vi "table test test.vi"() -> ()   [LabVIEW 2019]
uses:
  Ctrl/Table Save.ctl
  Ctrl/MeasureDisplayTab.ctl
  Ctrl/PD Table Save Low Index.ctl
  Ctrl/PD Table Save Col Index.ctl
  <vilib>/Utility/sysdir.llb/System Directory Type.ctl
  <vilib>/Utility/file.llb/Read Delimited Spreadsheet (string).vi
  <vilib>/Utility/file.llb/Write Delimited Spreadsheet (string).vi
panel:
  in  "SN":string="012345678911111111112"
  out "硬體":string
  out "Read SN Table":string[][](array[string])
  out "first row":string[](array[string])
  out "all rows":string[][](array[string])
  out "error out":errorcluster
  in  "Read SN Table 2":string[][](array[string])
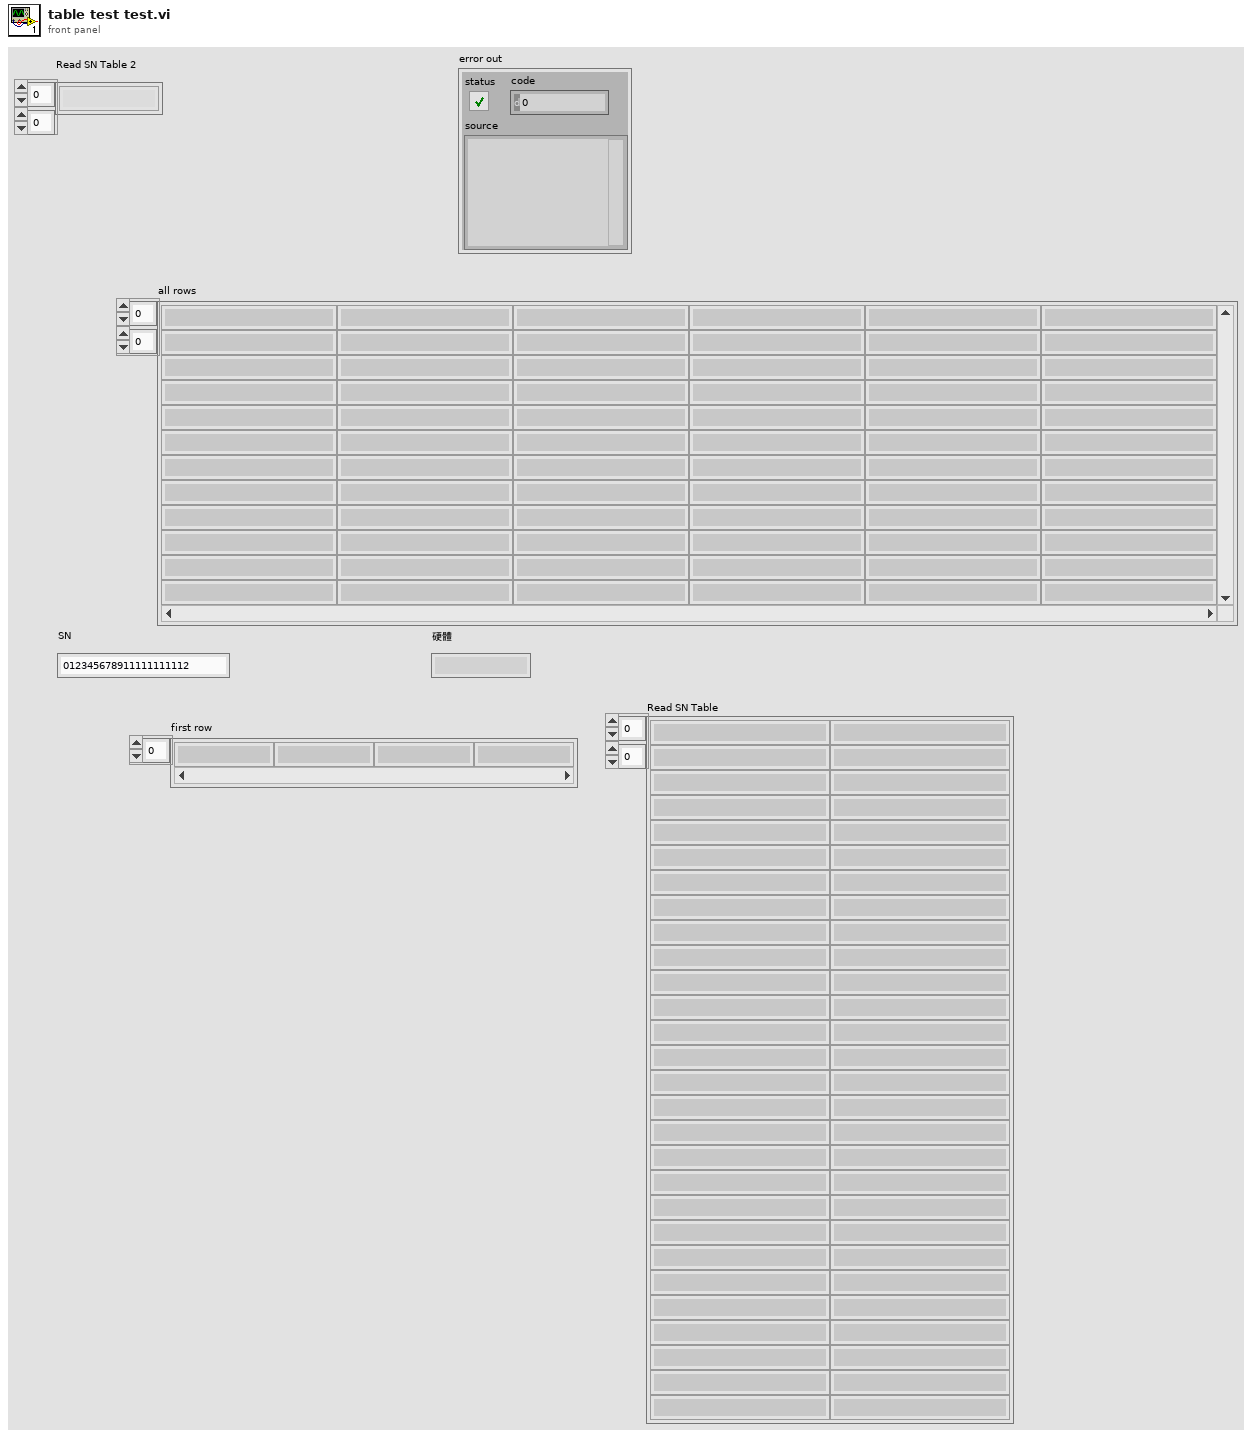
[diagram p1: front panel]
types:
  T1 = typedef "Table Save.ctl" = enum16{"initial", "Add", "Write", "Replace", "Delete", "REad", "RedTable", "Load"}
  T2 = typedef "MeasureDisplayTab.ctl" = enum16{"Tray Barcode", "PCBA BARCODE", "硬體(Tool初始化)", "company(Tool初始化)", "耗電流 uA(電流表)", "電池負載電壓", "晶片ID(Tool FORMAT)", "雷雕ID(TOOl scan、藍芽接收器)", "Format(Tool FORMAT)", "Programe(Tool Programe)", "MAC(藍芽接收器)", "ID(藍芽接收器)", "KPA(藍芽接收器)", "溫度(藍芽接收器)", "SENSOR電池電壓(藍芽接收器)", "RSSI(藍芽接收器)", "SensorType_315(FSK scan)", "FSKsnVol_315(FSK scan)", "FSKscanl_315(FSK scan)", "P_315(FSK scan)", "T_315(FSK scan)", "SensorType_433(ASK scan)", "ASKsnVol_433(ASK scan)", "ASKscan_433(ASK scan)", "P_433(ASK scan)", "T_433(ASK scan)", "測高Data"}
  T3 = typedef "PD Table Save Col Index.ctl" = enum16{"Col A", "Col B", "PCBA SN_C", "scan 半成品 ID_1_D", "半成品 Waste_Time_E", "半成品 Result_F", "半成品 DateTime_G", "433半成品 版本_H", "433半成品 company_I", "433半成品 FF_J", "433半成品 SensorType_K", "433半成品 BattVol_L", "433半成品 ASKsnVOL_M", "433半成品 ID_2_N", "433半成品 Format_O", "433半成品 Programe_P", "433半成品 ASKscan_Q", "433半成品 FSKscan_R", "433半成品 Batt_S", "433半成品 SN_T", "433半成品 Ptest_U", "433半成品 Ttest_V", "433半成品 P_W", "433半成品 T_X", "433半成品 結果_Y", "433半成品 箱號_Z", "不良代碼_AA", "電流_AB", "電池電壓_AC", "315半成品 版本_AD", "315半成品 company_AE", "315半成品 FF_AF", "315半成品 SensorType_AG", "315半成品 BattVol_AH", "315半成品 ASKsnVOL_AI", "315半成品 ID_2_AJ", "315半成品 Format_AK", "315半成品 Programe_AL", "315半成品 ASKscan_AM", "315半成品 FSKscan_AN", "315半成品 Batt_AO", "315半成品 SN_AP", "315半成品 Ptest_AQ", "315半成品 Ttest_AR", "315半成品 P_AS", "315半成品 T_AT"}
  T4 = typedef "PD Table Save Low Index.ctl" = enum16{"low 1", "low 2", "low 3", "low 4", "一般模式F", "一般模式P", "一般模式S", "low 8", "藍芽模式F", "藍芽模式P", "藍芽模式S"}
  T5 = typedef "System Directory Type.ctl" = i32
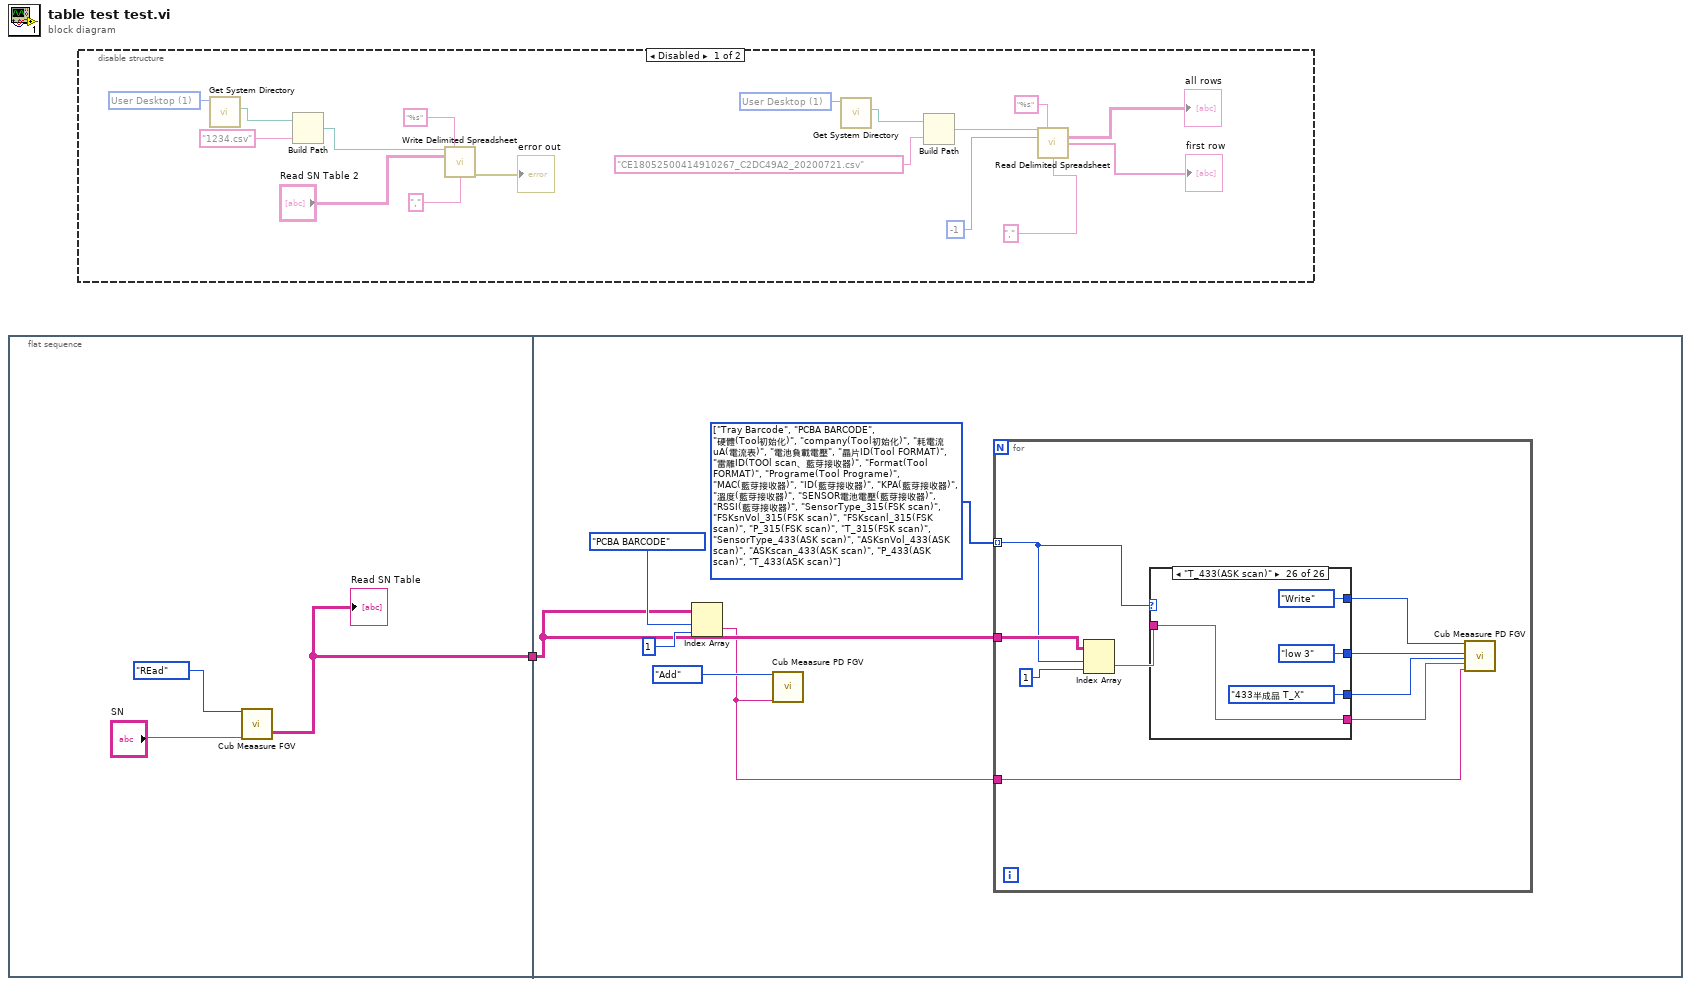
[diagram p0: block diagram]
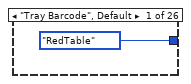
[diagram p3: hidden frame]
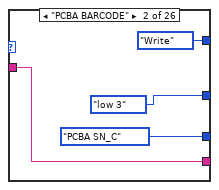
[diagram p4: hidden frame]
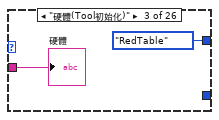
[diagram p5: hidden frame]
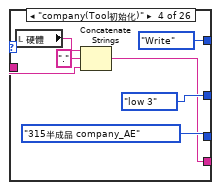
[diagram p6: hidden frame]
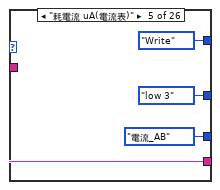
[diagram p7: hidden frame]
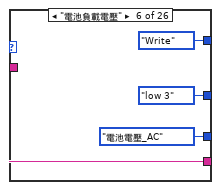
[diagram p8: hidden frame]
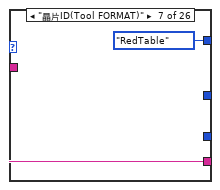
[diagram p9: hidden frame]
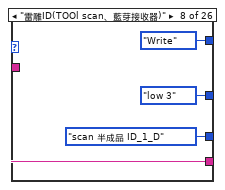
[diagram p10: hidden frame]
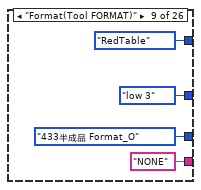
[diagram p11: hidden frame]
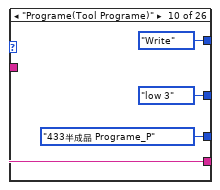
[diagram p12: hidden frame]
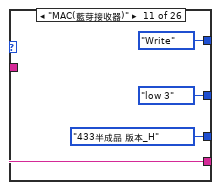
[diagram p13: hidden frame]
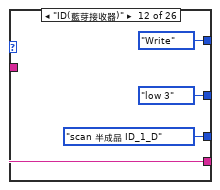
[diagram p14: hidden frame]
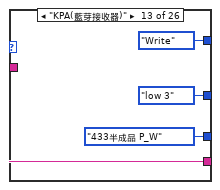
[diagram p15: hidden frame]
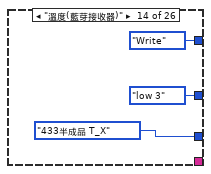
[diagram p16: hidden frame]
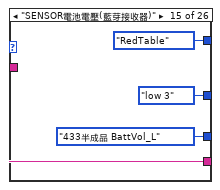
[diagram p17: hidden frame]
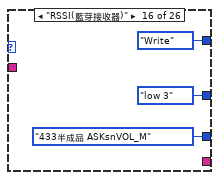
[diagram p18: hidden frame]
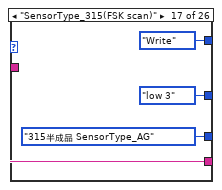
[diagram p19: hidden frame]
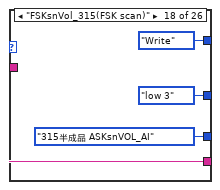
[diagram p20: hidden frame]
diagram:
  n1 = flat-sequence {
    tunnel: [w3] -> w1
    tunnel: w1 -> [w7]
    frame #0 {
      n2 = call "Cub Meaasure FGV.vi"("Action"=Table_Save."REad", "SN"="SN") -> ("Read SN Table"=w3:string[][])  [unwired: 10 in, 7 out]
      "Read SN Table" <- w3
    }
    frame #1 {
      w5 = T2[] [enum."Tray Barcode", enum."PCBA BARCODE", enum."硬體(Tool初始化)", enum."company(Tool初始化)", enum."耗電流 uA(電流表)", enum."電池負載電壓", enum."晶片ID(Tool FORMAT)", enum."雷雕ID(TOOl scan、藍芽接收器)", enum."Format(Tool FORMAT)", enum."Programe(Tool Programe)", enum."MAC(藍芽接收器)", enum."ID(藍芽接收器)", enum."KPA(藍芽接收器)", enum."溫度(藍芽接收器)", enum."SENSOR電池電壓(藍芽接收器)", enum."RSSI(藍芽接收器)", enum."SensorType_315(FSK scan)", enum."FSKsnVol_315(FSK scan)", enum."FSKscanl_315(FSK scan)", enum."P_315(FSK scan)", enum."T_315(FSK scan)", enum."SensorType_433(ASK scan)", enum."ASKsnVol_433(ASK scan)", enum."ASKscan_433(ASK scan)", enum."P_433(ASK scan)", enum."T_433(ASK scan)"] items=["Tray Barcode", "PCBA BARCODE", "硬體(Tool初始化)", "company(Tool初始化)", "耗電流 uA(電流表)", "電池負載電壓", "晶片ID(Tool FORMAT)", "雷雕ID(TOOl scan、藍芽接收器)", "Format(Tool FORMAT)", "Programe(Tool Programe)", "MAC(藍芽接收器)", "ID(藍芽接收器)", "KPA(藍芽接收器)", "溫度(藍芽接收器)", "SENSOR電池電壓(藍芽接收器)", "RSSI(藍芽接收器)", "SensorType_315(FSK scan)", "FSKsnVol_315(FSK scan)", "FSKscanl_315(FSK scan)", "P_315(FSK scan)", "T_315(FSK scan)", "SensorType_433(ASK scan)", "ASKsnVol_433(ASK scan)", "ASKscan_433(ASK scan)", "P_433(ASK scan)", "T_433(ASK scan)", "測高Data"]
      n3 = Index Array(array=w7, index (row)=MeasureDisplayTab."PCBA BARCODE" ("Save Index"), index (col)=1 ("disabled index (col)")) -> (element=w6:string)
      n4 = call "Cub Meaasure PD FGV.vi"("Action"=Table_Save."Add", "SN"=w6) -> ()  [unwired: 10 in, 8 out]
      n5 = for {
        tunnel: w7 -> [w17]
        tunnel: w5 -> [w14] mode=indexing
        tunnel: w6 -> [w11]
        n6 = Index Array(array=w17, index (row)=w14, index (col)=1 ("disabled index (col)")) -> (element=w15:string)
        n7 = case shown="\"T_433(ASK scan)\"" w14 {
          tunnel: w15 -> [_ w22 w25 w28 w34 w38 w42 w44 _ w52 w56 w60 w64 _ w71 _ w78 w82 w86 w90 w94 w98 w102 w106 w110 w114]
          tunnel: [_ PD_Table_Save_Low_Index."low 3" _ PD_Table_Save_Low_Index."low 3" PD_Table_Save_Low_Index."low 3" PD_Table_Save_Low_Index."low 3" _ PD_Table_Save_Low_Index."low 3" PD_Table_Save_Low_Index."low 3" PD_Table_Save_Low_Index."low 3" PD_Table_Save_Low_Index."low 3" PD_Table_Save_Low_Index."low 3" PD_Table_Save_Low_Index."low 3" PD_Table_Save_Low_Index."low 3" PD_Table_Save_Low_Index."low 3" PD_Table_Save_Low_Index."low 3" PD_Table_Save_Low_Index."low 3" PD_Table_Save_Low_Index."low 3" PD_Table_Save_Low_Index."low 3" PD_Table_Save_Low_Index."low 3" PD_Table_Save_Low_Index."low 3" PD_Table_Save_Low_Index."low 3" PD_Table_Save_Low_Index."low 3" PD_Table_Save_Low_Index."low 3" PD_Table_Save_Low_Index."low 3" PD_Table_Save_Low_Index."low 3"] -> w19
          tunnel: [_ PD_Table_Save_Col_Index."PCBA SN_C" ("Save Col Index") _ PD_Table_Save_Col_Index."315半成品 company_AE" ("Save Col Index") PD_Table_Save_Col_Index."電流_AB" ("Save Col Index") PD_Table_Save_Col_Index."電池電壓_AC" ("Save Col Index") _ PD_Table_Save_Col_Index."scan 半成品 ID_1_D" ("Save Col Index") PD_Table_Save_Col_Index."433半成品 Format_O" ("Save Col Index") PD_Table_Save_Col_Index."433半成品 Programe_P" ("Save Col Index") PD_Table_Save_Col_Index."433半成品 版本_H" ("Save Col Index") PD_Table_Save_Col_Index."scan 半成品 ID_1_D" ("Save Col Index") PD_Table_Save_Col_Index."433半成品 P_W" ("Save Col Index") PD_Table_Save_Col_Index."433半成品 T_X" ("Save Col Index") PD_Table_Save_Col_Index."433半成品 BattVol_L" ("Save Col Index") PD_Table_Save_Col_Index."433半成品 ASKsnVOL_M" ("Save Col Index") PD_Table_Save_Col_Index."315半成品 SensorType_AG" ("Save Col Index") PD_Table_Save_Col_Index."315半成品 ASKsnVOL_AI" ("Save Col Index") PD_Table_Save_Col_Index."315半成品 FSKscan_AN" ("Save Col Index") PD_Table_Save_Col_Index."315半成品 P_AS" ("Save Col Index") PD_Table_Save_Col_Index."315半成品 T_AT" ("Save Col Index") PD_Table_Save_Col_Index."433半成品 SensorType_K" ("Save Col Index") PD_Table_Save_Col_Index."433半成品 ASKsnVOL_M" ("Save Col Index") PD_Table_Save_Col_Index."433半成品 ASKscan_Q" ("Save Col Index") PD_Table_Save_Col_Index."433半成品 P_W" ("Save Col Index") PD_Table_Save_Col_Index."433半成品 T_X" ("Save Col Index")] -> w18
          tunnel: [_ w22 _ w27 w34 w38 w42 w44 "NONE" w52 w56 w60 w64 _ w71 _ w78 w82 w86 w90 w94 w98 w102 w106 w110 w114] -> w12
          tunnel: [Table_Save."RedTable" ("Action") Table_Save."Write" ("Action") Table_Save."RedTable" ("Action") Table_Save."Write" ("Action") Table_Save."Write" ("Action") Table_Save."Write" ("Action") Table_Save."RedTable" ("Action") Table_Save."Write" ("Action") Table_Save."RedTable" ("Action") Table_Save."Write" ("Action") Table_Save."Write" ("Action") Table_Save."Write" ("Action") Table_Save."Write" ("Action") Table_Save."Write" ("Action") Table_Save."RedTable" ("Action") Table_Save."Write" ("Action") Table_Save."Write" ("Action") Table_Save."Write" ("Action") Table_Save."Write" ("Action") Table_Save."Write" ("Action") Table_Save."Write" ("Action") Table_Save."Write" ("Action") Table_Save."Write" ("Action") Table_Save."Write" ("Action") Table_Save."Write" ("Action") Table_Save."Write" ("Action")] -> w13
          frame "Tray Barcode", Default {
          }
          frame "PCBA BARCODE" {
          }
          frame "硬體(Tool初始化)" {
            "硬體" <- w25
          }
          frame "company(Tool初始化)" {
            n8 = local read "硬體"() -> (w30:string)
            n9 = Concatenate Strings(w30, "." ("string"), w28) -> (w27:string)
          }
          frame "耗電流 uA(電流表)" {
          }
          frame "電池負載電壓" {
          }
          frame "晶片ID(Tool FORMAT)" {
          }
          frame "雷雕ID(TOOl scan、藍芽接收器)" {
          }
          frame "Format(Tool FORMAT)" {
          }
          frame "Programe(Tool Programe)" {
          }
          frame "MAC(藍芽接收器)" {
          }
          frame "ID(藍芽接收器)" {
          }
          frame "KPA(藍芽接收器)" {
          }
          frame "溫度(藍芽接收器)" {
          }
          frame "SENSOR電池電壓(藍芽接收器)" {
          }
          frame "RSSI(藍芽接收器)" {
          }
          frame "SensorType_315(FSK scan)" {
          }
          frame "FSKsnVol_315(FSK scan)" {
          }
          frame "FSKscanl_315(FSK scan)" {
          }
          frame "P_315(FSK scan)" {
          }
          frame "T_315(FSK scan)" {
          }
          frame "SensorType_433(ASK scan)" {
          }
          frame "ASKsnVol_433(ASK scan)" {
          }
          frame "ASKscan_433(ASK scan)" {
          }
          frame "P_433(ASK scan)" {
          }
          frame "T_433(ASK scan)" {
          }
        }
        n10 = call "Cub Meaasure PD FGV.vi"("Action"=w13, "Save low Index"=w19, "Save Col Index"=w18, "DataIn"=w12, "SN"=w11) -> ()  [unwired: 7 in, 8 out]
      }
    }
  }
  n11 = disable-structure shown="Disabled" {
    frame Disabled {
      w121 = T5 1 items=["User Home"=0, "User Desktop"=1, "User Documents"=2, "User Application Data"=3, "User Preferences"=4, "User Temporary"=5, "Public Documents"=6, "Public Application Data"=7, "Public Preferences"=8, "Public Cache"=13, "System Core Libraries"=9, "System Installed Libraries"=10, "Application Files"=11, "Boot Volume Root"=12] ("system directory type")
      w130 = T5 1 items=["User Home"=0, "User Desktop"=1, "User Documents"=2, "User Application Data"=3, "User Preferences"=4, "User Temporary"=5, "Public Documents"=6, "Public Application Data"=7, "Public Preferences"=8, "Public Cache"=13, "System Core Libraries"=9, "System Installed Libraries"=10, "Application Files"=11, "Boot Volume Root"=12] ("system directory type")
      n12 = call <vilib>:"Get System Directory.vi"("system directory type"=w130) -> ("system directory"=w133:path)  [unwired: 10 in]
      n13 = Build Path(base path=w133, name or relative path="1234.csv") -> (appended path=w134:path)
      n14 = call-poly <vilib>:"Write Delimited Spreadsheet.vi"("file path (dialog if empty)"=w134, "format (%s)"="%s", "2D data"="Read SN Table 2", "delimiter (\\t)"="," ("delimiter (\\t)")) -> ("error out"=→"error out":errorcluster)  [unwired: 10 in, 1 out]
      n15 = call <vilib>:"Get System Directory.vi"("system directory type"=w121) -> ("system directory"=w120:path)  [unwired: 10 in]
      n16 = Build Path(base path=w120, name or relative path="CE18052500414910267_C2DC49A2_20200721.csv") -> (appended path=w119:path)
      n17 = call-poly <vilib>:"Read Delimited Spreadsheet.vi"("file path (dialog if empty)"=w119, "format (%s)"="%s", "number of rows (all:-1)"=-1, "delimiter (\\t)"="," ("delimiter (\\t)")) -> ("all rows"=→"all rows":string[][], "first row"=→"first row":string[])  [unwired: 6 in, 4 out]
    }
    frame Enabled {
    }
  }
